vi "summariseStringArray.vi"(10 "stringArray":string[](array[string])) -> (1 "firstSingleMostCommon":string, 3 "percentagesString":string)   [LabVIEW 2022 SP3]
uses:
  c5fd07db-b153-df44-8ee8-7e7effe9a91e.vi
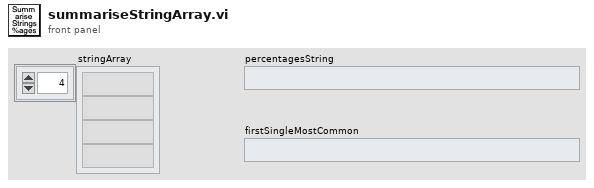
[diagram p1: front panel]
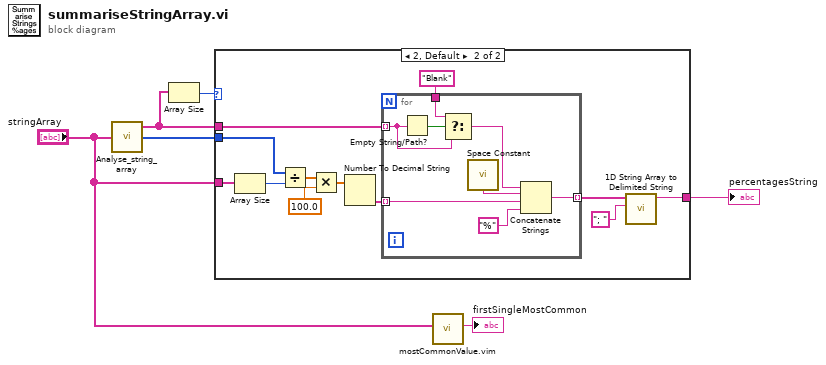
[diagram p0: block diagram]
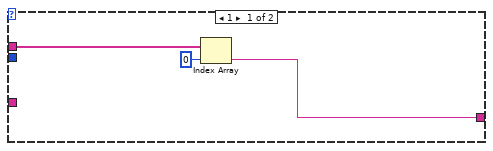
[diagram p2: hidden frame]
diagram:
  n1 = call "Analyse_string_array.vi"("String array"="stringArray") -> ("Unique strings"=w5:string[], "Frequency"=w4:i32[])  [unwired: 1 out]
  n2 = Array Size(array=w5) -> (size(s)=w6:i32)
  n3 = case shown="2, Default" w6 {
    tunnel: [w8 w11] -> w3
    tunnel: w4 -> [_ w17]
    tunnel: w5 -> [w7 w16]
    tunnel: "stringArray" -> [_ w13]
    frame 1 {
      n4 = Index Array(array=w7, index=0) -> (element=w8:string)
    }
    frame 2, Default {
      n5 = Array Size(array=w13) -> (size(s)=w14:i32)
      n6 = Divide(x=w17, y=w14) -> (x/y=w21:dbl[])
      n7 = Multiply(x=w21, y=100.0) -> (x*y=w19:dbl[])
      n8 = Number To Decimal String(number=w19) -> (decimal integer string=w18:string[])  [unwired: 1 out]
      n9 = for {
        tunnel: w18 -> [w29] mode=indexing
        tunnel: w16 -> [w25] mode=indexing
        tunnel: "Blank" -> [w27]
        tunnel: [w22] -> w12 mode=indexing
        n10 = Empty String/Path?(string/path=w25) -> (empty?=w26:bool)
        n11 = Select(t=w27, s=w26, f=w25) -> (s? t:f=w24:string)
        n12 = call <vilib>:"Space Constant.vi"() -> ("String"=w28:string)
        n13 = Concatenate Strings(w24, w28, w29, "%") -> (w22:string)
      }
      n14 = call <vilib>:"1D String Array to Delimited String.vi"("delimiter"="; ", "string array"=w12) -> ("delimited string"=w11:string)  [unwired: 9 in]
    }
  }
  "percentagesString" <- w3
  n15 = call "mostCommonValue.vim"("arrayIn"="stringArray") -> ("mode"=→"firstSingleMostCommon":string)  [unwired: 8 in, 2 out]
